vi "Main.vi"() -> ()   [LabVIEW 2021]
uses:
  <vilib>/FPGAPlugInAG/myRIO-1900/niLvFpga_Open_myRIO-1900.vi
  <vilib>/rvi/interface/common/dynamic/niFpgaDynamicAddResources.vi
  <vilib>/measure/macond.llb/IIR Filter for 1 Chan.vi
  <vilib>/FPGAPlugInAG/Dynamic/niLvFpga_Close_Dynamic.vi
  <vilib>/rvi/interface/nirviOpenFPGA/nirviOpenFPGA.xnode
  FPGA Bitfiles/FPGA Audio Streaming (with LEDs).lvbitx
  FPGA Audio Streaming.vi
  <vilib>/rvi/interface/nirviCloseFPGA/nirviCloseFPGA.xnode
  <vilib>/measure/NI_MAPro.lvlib
panel:
  in  "IIR filter specifications":T1={"Topology"=enum."Inverse Chebyshev", "Type"=enum."Lowpass", "Order"=10, "Fc1"=100.0, "Fc2"=200.0, "PB Ripple"=1.0, "SB Attenuation"=60.0} {"SB Attenuation" format="%#.6g"; "PB Ripple" format="%#.6g"; "Fc2" format="%#.6g"; "Fc1" format="%#.6g"}
  out "Real-Time Raw Audio":waveform(i16)(graph)
  out "Sample Rate [Hz]":dbl=44101.0
  out "Magnitude response":cluster{"f0":dbl, "df":dbl, "Mag H(w)":dbl[]}(graph)={"f0"=0.0, "df"=0.9765625, "Mag H(w)"=[]}
  out "Phase response":cluster{"f0":dbl, "df":dbl, "Phase H(w)":dbl[]}(graph)={"f0"=0.0, "df"=0.9765625, "Phase H(w)"=[]}
  in  "Volume":dbl(slide)=1.0 scale=0.0..1.0
  out "Raw vs. Filtered Audio Spectrum":dynamicdata(graph)
  in  "stop":bool
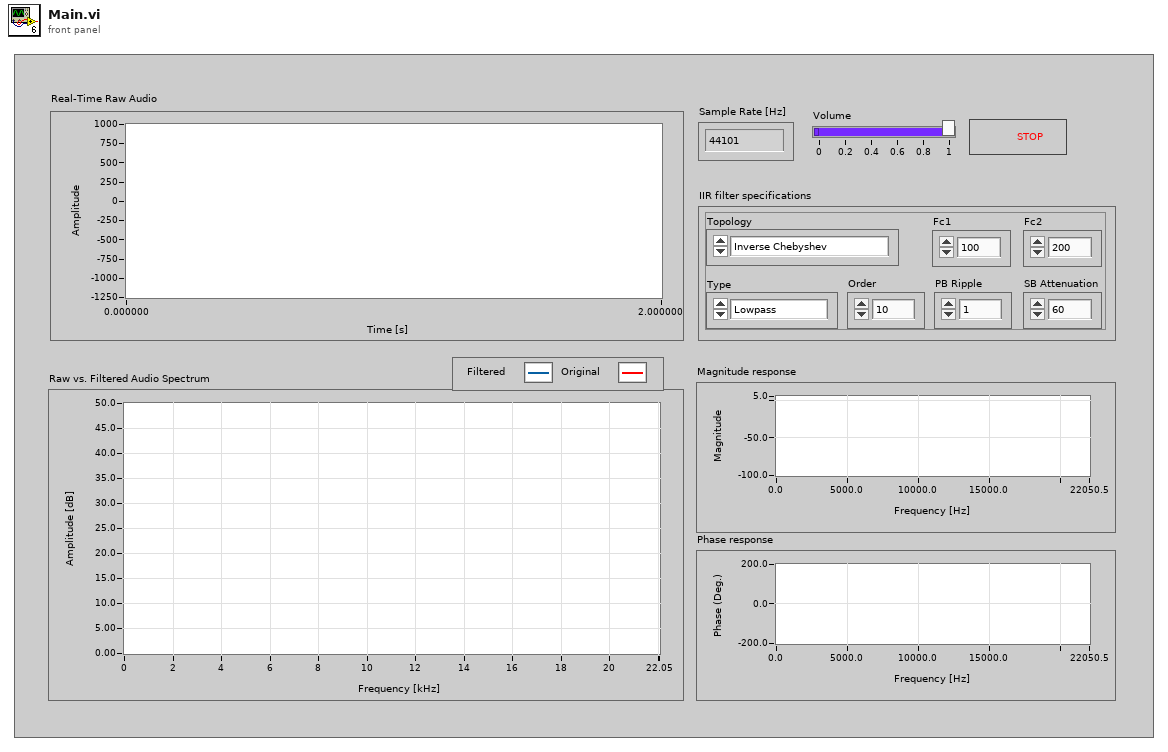
[diagram p1: front panel]
types:
  T1 = cluster{"Topology":enum16{"Off", "Butterworth", "Chebyshev", "Inverse Chebyshev", "Elliptic", "Bessel"}, "Type":enum16{"Lowpass", "Highpass", "Bandpass", "Bandstop"}, "Order":i32, "Fc1":dbl, "Fc2":dbl, "PB Ripple":dbl, "SB Attenuation":dbl}
  T2 = enum16{"FFT spectrum", "Power spectrum", "Cross spectrum", "Frequency response"}
  T3 = cluster{"magnitude H(w)":cluster{"f0":dbl, "df":dbl, "Mag H(w)":dbl[]}, "phase H(w)":cluster{"f0":dbl, "df":dbl, "Phase H(w)":dbl[]}, "order":i32}
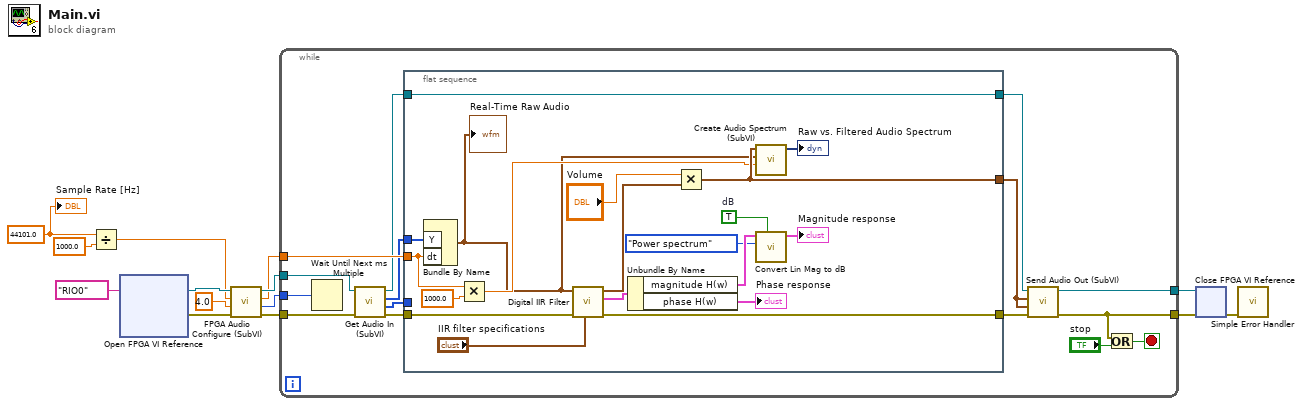
[diagram p0: block diagram]
diagram:
  w3 = 44101.0 ("Sample Rate (kHz)")
  n1 = Divide(x=w3, y=1000.0) -> (x/y=w1:dbl)
  n2 = xnode "Open FPGA VI Reference"("resource name"=tag "RIO0") -> ("FPGA VI Reference Out"=w7:refnum<k20>, "error out"=w14:errorcluster)  [unwired: 1 in]
  n3 = call "FPGA Audio Configure (SubVI).vi"("error in (no error)"=w14, "Read Rate (Hz)"=4.0, "Audio Sample Rate (kHz)"=w1, "Refnum in"=w7) -> ("error out"=w9:errorcluster, "Required loop period (ms)"=w5:u32, "Audio dt (ms)"=w6:dbl, "Refnum out"=w13:refnum<k20>)  [unwired: 4 in]
  n4 = while {
    tunnel: w13 -> [w26]
    tunnel: [w25] -> w12
    tunnel: [w21] -> w11
    tunnel: w5 -> [w15]
    tunnel: w9 -> [w27]
    tunnel: w6 -> [w24]
    stop <- w28 stop-if-true
    n5 = Wait Until Next ms Multiple(millisecond multiple=w15) -> ()  [unwired: 1 out]
    n6 = call "Get Audio In (SubVI).vi"("error in (no error)"=w27, "Refnum in"=w26) -> ("error out"=w19:errorcluster, "Right Audio In"=w16:i16[], "Left Audio In"=w22:i16[], "Refnum out"=w20:refnum<k20>)  [unwired: 6 in]
    n7 = flat-sequence {
      tunnel: w24 -> [w33]
      tunnel: [w46] -> w23
      tunnel: w22 -> [w31]
      tunnel: w20 -> [w43]
      tunnel: w19 -> [w37]
      tunnel: [w43] -> w18
      tunnel: [w36] -> w17
      tunnel: w16 -> [_]
      frame #0 {
        w41 = TRUE  # dB
        n8 = Bundle By Name("Y"=w31, "dt"=w33) -> (w30:waveform(i16))  [unwired: 1 in]
        "Real-Time Raw Audio" <- w30
        n9 = Multiply(x=w33, y=1000.0) -> (x*y=w32:dbl)
        n10 = call-poly <vilib>:"Digital IIR Filter.vi"("IIR filter specifications"="IIR filter specifications", "error in (no error)"=w37, "signal in"=w30) -> ("error out"=w36:errorcluster, "filter information"=w35:T3, "signal out"=w34:waveform(dbl))  [unwired: 6 in]
        n11 = Unbundle By Name(w35) -> ("magnitude H(w)"=w40:cluster{"f0":dbl, "df":dbl, "Mag H(w)":dbl[]}, "phase H(w)"=→"Phase response":cluster{"f0":dbl, "df":dbl, "Phase H(w)":dbl[]})
        n12 = Multiply(x="Volume", y=w34) -> (x*y=w46:waveform(dbl))
        n13 = call "Create Audio Spectrum (SubVI).vi"("Sample Period (ms)"=w32, "Raw Audio"=w30, "Filtered Audio"=w46) -> ("FFT Out"=→"Raw vs. Filtered Audio Spectrum":dynamicdata)  [unwired: 8 in]
        n14 = call "Convert Lin Mag to dB.vi"("convert to dB"=w41, "spectrum type"=T2."Power spectrum", "magnitude H(w)"=w40) -> ("magnitude H(w) in dB"=→"Magnitude response":cluster{"f0":dbl, "df":dbl, "Mag H(w)":dbl[]})  [unwired: 8 in]
      }
    }
    n15 = call "Send Audio Out (SubVI).vi"("error in (no error)"=w17, "Right Audio Out"=w23, "Left Audio Out"=w23, "Refnum in"=w18) -> ("error out"=w21:errorcluster, "Refnum out"=w25:refnum<k20>)  [unwired: 6 in]
    n16 = Or(x=w21, y="stop") -> (x .or. y?=w28:bool)
  }
  n17 = xnode "Close FPGA VI Reference"("FPGA VI Reference In"=w12, "error in"=w11) -> ("error out"=w4:errorcluster)
  n18 = call <vilib>:"Simple Error Handler.vi"("error in (no error)"=w4) -> ()  [unwired: 4 in, 5 out]
  "Sample Rate [Hz]" <- w3
